vi "Include SDI SSM and Parity Parameters.vi"(8 "create SDI (F)":bool, 9 "create SSM (F)":bool, 10 "create parity (F)":bool, 11 "parameters":T1[](array[typedef])) -> (3 "parameters out":T1[](array[typedef]))   [LabVIEW 2020, in "Ballard ARINC 429 Scripting.lvlib"]
uses:
  Ballard ARINC 429 Scripting.lvlib
  Encoding and Decoding/Encoding.ctl
  Encoding and Decoding/Encoding and Decoding.lvlib
  Shared/Parameter Definition.ctl
  Shared/Direction.ctl
  Shared/VS Channel Definition for Parameter.ctl
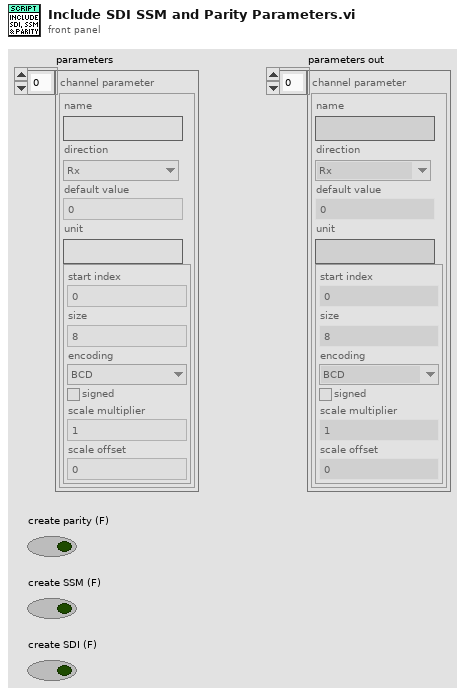
[diagram p1: front panel]
types:
  T1 = typedef "VS Channel Definition for Parameter.ctl" = cluster{"name":string, "direction":T2, "default value":dbl, "unit":string, "Parameter":T3}
  T2 = typedef "Direction.ctl" = enum16{"Rx", "Tx"}
  T3 = typedef "Parameter Definition.ctl" = cluster{"start index":i32, "size":i32, "encoding":T4, "signed":bool, "scale multiplier":dbl, "scale offset":dbl}
  T4 = typedef "Encoding and Decoding.lvlib/Encoding.ctl" = enum16{"BNR", "BCD", "Discrete"}
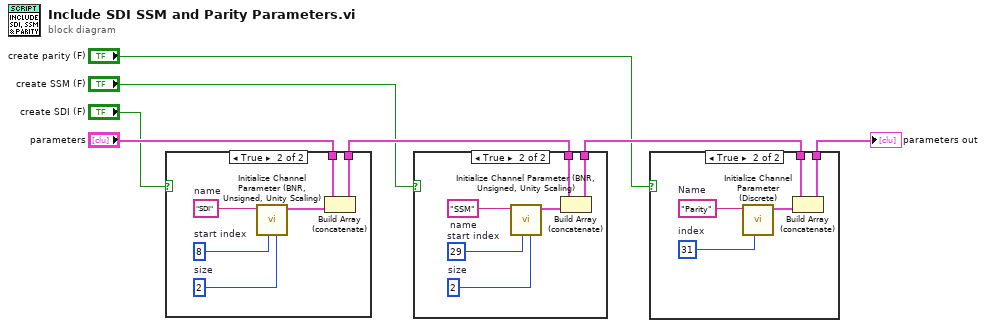
[diagram p0: block diagram]
diagram:
  n1 = case shown="True" "create SDI (F)" {
    tunnel: "parameters" -> [w8 w14]
    tunnel: [w8 w13] -> w5
    frame False {
    }
    frame True {
      w12 = 2  # size
      w11 = 8  # start index
      w10 = "SDI"  # name
      n2 = call "Initialize Channel Parameter (BNR, Unsigned, Unity Scaling).vi"("size"=w12, "start index"=w11, "name"=w10) -> ("channel parameter"=w9:T1)  [unwired: 8 in]
      n3 = Build Array (concatenate)(w14, w9) -> (w13:T1[])
    }
  }
  n4 = case shown="True" "create SSM (F)" {
    tunnel: w5 -> [w15 w21]
    tunnel: [w15 w20] -> w3
    frame False {
    }
    frame True {
      w17 = 2  # size
      w18 = 29  # start index
      w19 = "SSM"  # name
      n5 = call "Initialize Channel Parameter (BNR, Unsigned, Unity Scaling).vi"("size"=w17, "start index"=w18, "name"=w19) -> ("channel parameter"=w16:T1)  [unwired: 8 in]
      n6 = Build Array (concatenate)(w21, w16) -> (w20:T1[])
    }
  }
  n7 = case shown="True" "create parity (F)" {
    tunnel: w3 -> [w22 w27]
    tunnel: [w22 w26] -> w2
    frame False {
    }
    frame True {
      w23 = 31  # index
      w24 = "Parity"  # Name
      n8 = call "Initialize Channel Parameter (Discrete).vi"("index"=w23, "name"=w24) -> ("channel parameter"=w25:T1)  [unwired: 9 in]
      n9 = Build Array (concatenate)(w27, w25) -> (w26:T1[])
    }
  }
  "parameters out" <- w2
